vi "Zip up measurement definition.vi"(8 "error in (no error)":errorcluster, 10 "Measurement Name":string, 11 "class path":path) -> (0 "error out":errorcluster, 2 "output path":path)   [LabVIEW 2026, in "Server Controller.lvlib" / "Server Controller.lvclass"]
uses:
  Server Controller.lvclass
  Server Controller.lvclass/Server Controller.ctl
  <vilib>/Utility/sysdir.llb/System Directory Type.ctl
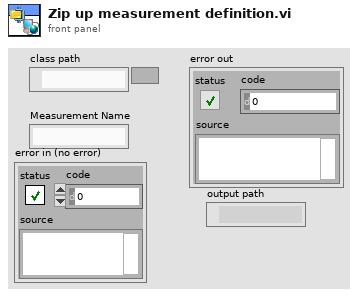
[diagram p1: front panel]
types:
  T1 = typedef "System Directory Type.ctl" = i32
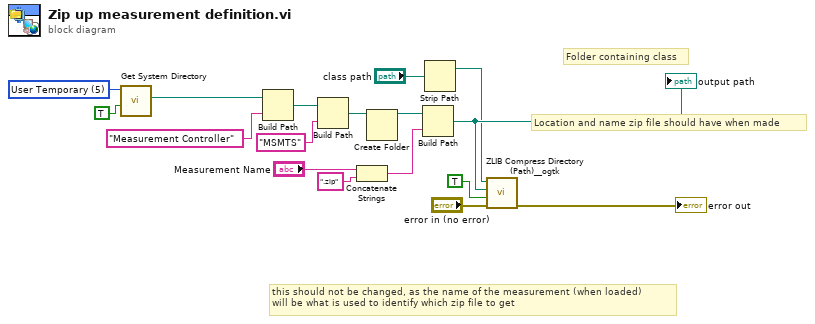
[diagram p0: block diagram]
diagram:
  w15 = T1 5 items=["User Home"=0, "User Desktop"=1, "User Documents"=2, "User Application Data"=3, "User Preferences"=4, "User Temporary"=5, "Public Documents"=6, "Public Application Data"=7, "Public Preferences"=8, "Public Cache"=13, "System Core Libraries"=9, "System Installed Libraries"=10, "Application Files"=11, "Boot Volume Root"=12] ("system directory type")
  # "this should not be changed, as the name of the measurement (when loaded)\nwill be what is used to identify which zip file to get"
  # "Location and name zip file should have when made"
  # "Folder containing class"
  n1 = call <vilib>:"Get System Directory.vi"("create directory if not found? (F)"=TRUE, "system directory type"=w15) -> ("system directory"=w13:path)  [unwired: 9 in]
  n2 = Build Path(base path=w13, name or relative path="Measurement Controller") -> (appended path=w11:path)
  n3 = Build Path(base path=w11, name or relative path="MSMTS") -> (appended path=w10:path)
  n4 = Concatenate Strings("Measurement Name", ".zip" ("string")) -> (w7:string)
  n5 = Create Folder(path (use dialog)=w10) -> (created path=w16:path)  [unwired: 2 in, 2 out]
  n6 = Build Path(base path=w16, name or relative path=w7) -> (appended path=w5:path)
  "output path" <- w5
  n7 = Strip Path(path="class path") -> (stripped path=w3:path)  [unwired: 1 out]
  n8 = call <userlib>:"ZLIB Compress Directory (Path)__ogtk.vi"("error in (no error)"="error in (no error)", "include subdirectories (F)"=TRUE, "archive name (root directory with .zip ending)"=w5, "root directory (file dialog)"=w3) -> ("error out"=→"error out":errorcluster)  [unwired: 5 in, 2 out]
